vi "ABFImport_Close.vi"(8 "error in (no error)":errorcluster, 11 "reference number":i32) -> (0 "error out":errorcluster)   [LabVIEW 2017]
uses:
  LV_ABFIO.dll
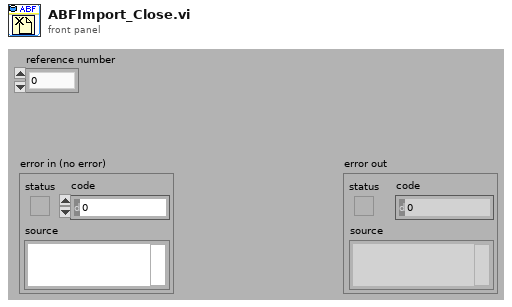
[diagram p1: front panel]
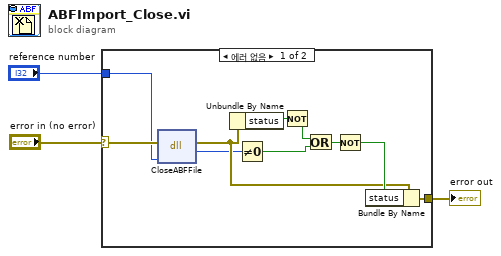
[diagram p0: block diagram]
diagram:
  n1 = case shown="에러 없음" "error in (no error)" {
    selector: "error in (no error)" -> [w7 w14]
    tunnel: [w8 w14] -> w2
    tunnel: "reference number" -> [w4 _]
    frame No Error {
      n2 = dll-call lib="C:/Users/KimYG/Application/Solution Package/APIs/LV_ABFIO.dll" fn="CloseABFFile"(error in=w7, "arg3"=w4) -> (error out=w6:errorcluster, "return type"=w5:i32)  [unwired: 3 in, 1 out]
      n3 = Unbundle By Name(w6) -> ("status"=w13:bool)
      n4 = Not Equal To 0?(x=w5) -> (x != 0?=w11:bool)
      n5 = Not(x=w13) -> (.not. x?=w12:bool)
      n6 = Or(x=w12, y=w11) -> (x .or. y?=w10:bool)
      n7 = Not(x=w10) -> (.not. x?=w9:bool)
      n8 = Bundle By Name(cluster=w6, "status"=w9) -> (w8:errorcluster)
    }
    frame Error {
    }
  }
  "error out" <- w2
